vi "Test akwizycji AI Enk.vi"() -> ()   [LabVIEW 2014]
uses:
  <vilib>/DAQmx/create/channels.llb/DAQmx Create Channel (CI-Position-Linear Encoder).vi
  <vilib>/DAQmx/create/channels.llb/DAQmx Create Channel (AI-Voltage-Basic).vi
  <vilib>/DAQmx/configure/timing.llb/DAQmx Timing (Sample Clock).vi
  <vilib>/DAQmx/read.llb/DAQmx Read (Counter 1D DBL 1Chan NSamp).vi
  <vilib>/DAQmx/read.llb/DAQmx Read (Analog 1D Wfm NChan NSamp).vi
panel:
  out "Waveform Graph":waveform(dbl)[](graph)
  in  "error in":errorcluster
  in  "stop":bool
  out "data":dbl[](array[numeric]) format="%#_6p"
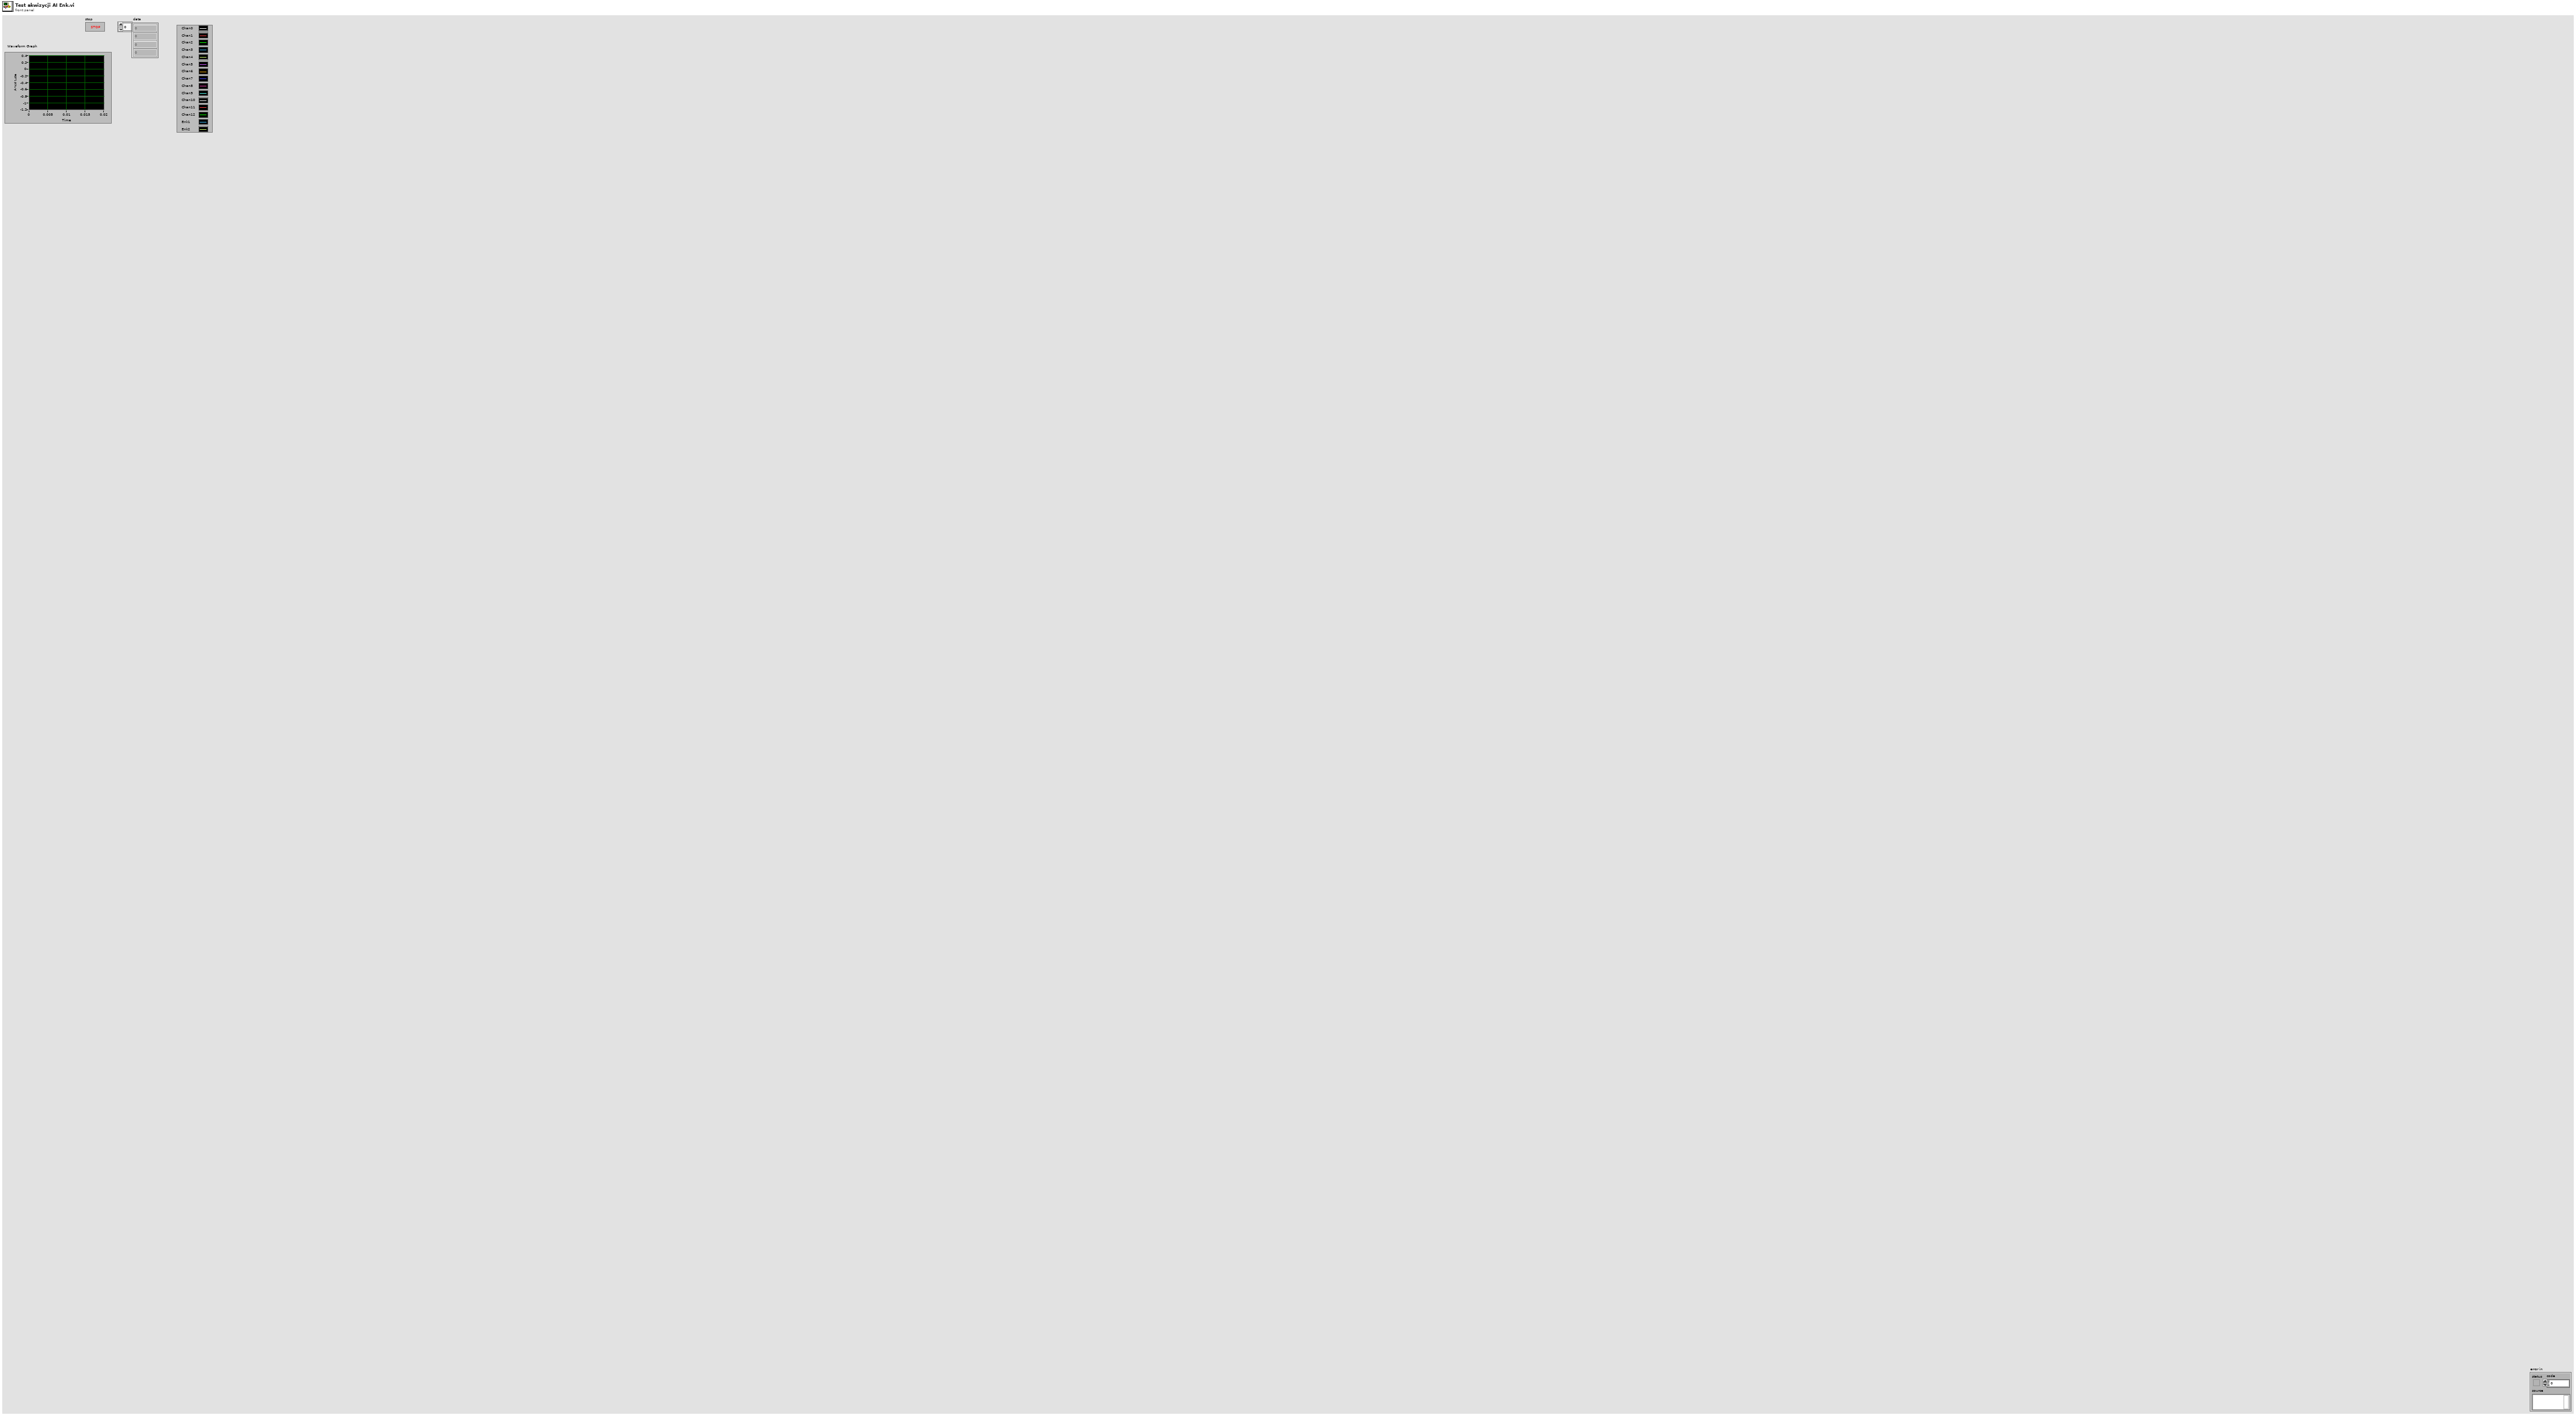
[diagram p1: front panel]
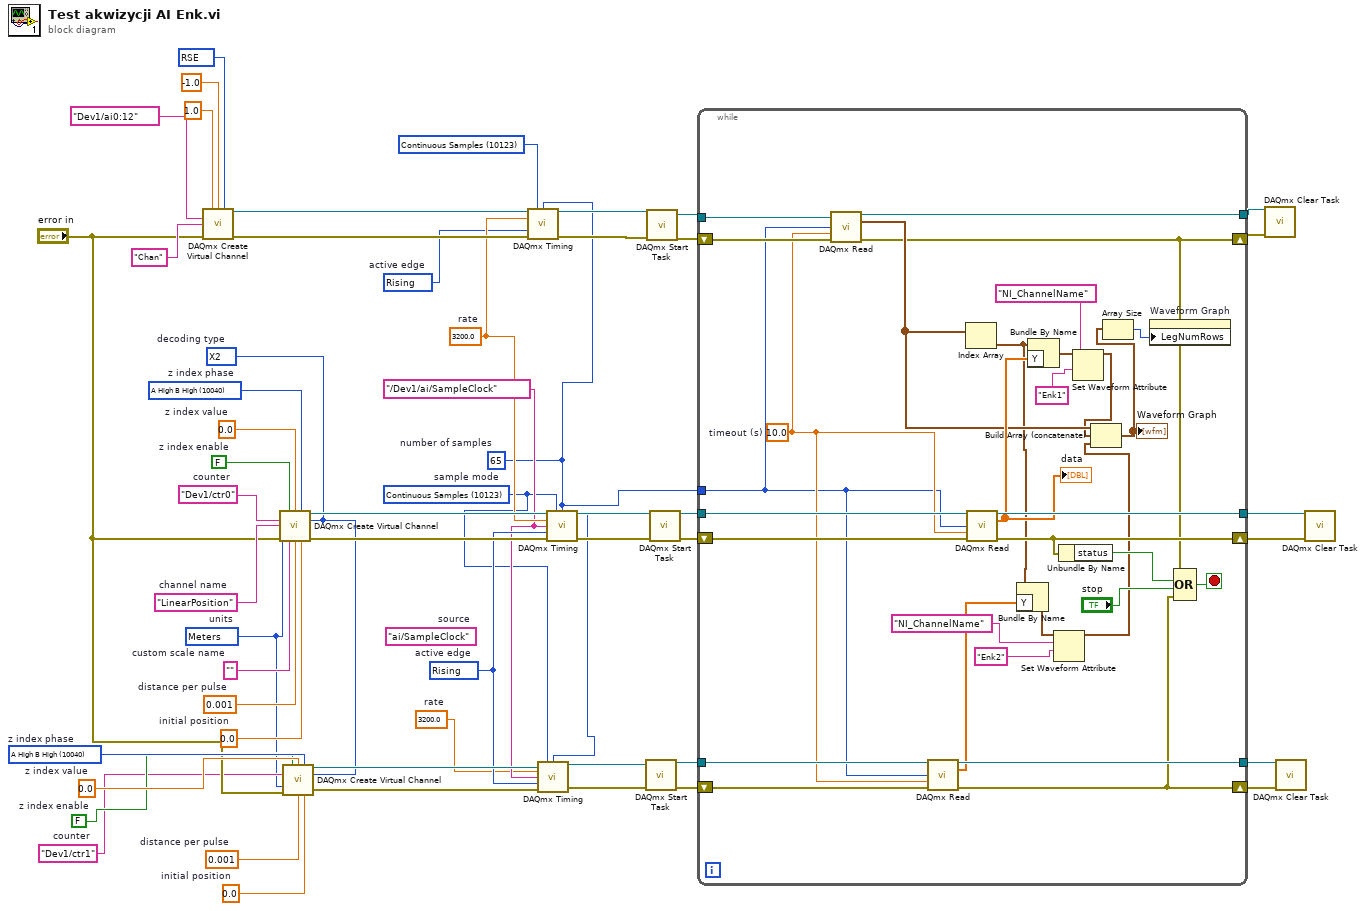
[diagram p0: block diagram]
diagram:
  w5 = 0.0  # initial position
  w6 = 0.001  # distance per pulse
  w12 = 10040 items=["A High B High"=10040, "A High B Low"=10041, "A Low B High"=10042, "A Low B Low"=10043]  # z index phase
  w11 = 0.0  # z index value
  w10 = FALSE  # z index enable
  w8 = "Dev1/ctr1"  # counter
  w15 = 3200.0  # rate
  w25 = 10280 items=["Rising"=10280, "Falling"=10171]  # active edge
  w27 = 10123 items=["Finite Samples"=10178, "Continuous Samples"=10123, "Hardware Timed Single Point"=12522] ("sample mode")
  w16 = tag "/Dev1/ai/SampleClock" ("source")
  w36 = 10083 items=["default"=-1, "RSE"=10083, "NRSE"=10078, "Differential"=10106, "Pseudodifferential"=12529] ("input terminal configuration")
  w13 = 10123 items=["Finite Samples"=10178, "Continuous Samples"=10123, "Hardware Timed Single Point"=12522]  # sample mode
  w26 = 3200.0  # rate
  w17 = 10280 items=["Rising"=10280, "Falling"=10171]  # active edge
  (unwired) "ai/SampleClock"  # source
  w14 = 65  # number of samples
  w7 = 10219 items=["Meters"=10219, "Inches"=10379, "Ticks"=10304, "From Custom Scale"=10065]  # units
  w18 = 10091 items=["X1"=10090, "X2"=10091, "X4"=10092, "Two Pulse Counting"=10313]  # decoding type
  w49 = 0.0  # initial position
  w48 = 0.001  # distance per pulse
  w46 = ""  # custom scale name
  w47 = 10040 items=["A High B High"=10040, "A High B Low"=10041, "A Low B High"=10042, "A Low B Low"=10043]  # z index phase
  w45 = 0.0  # z index value
  w44 = FALSE  # z index enable
  w43 = "LinearPosition"  # channel name
  w41 = "Dev1/ctr0"  # counter
  n1 = call-poly <vilib>:"DAQmx Create Virtual Channel.vi"("maximum value"=1.0, "minimum value"=-1.0, "input terminal configuration"=w36, "physical channels"=tag "Dev1/ai0:12", "name to assign"="Chan", "error in"="error in") -> ("task out"=w28:refnum<k21>, "error out"=w29:errorcluster)  [unwired: 8 in]
  n2 = call-poly <vilib>:"DAQmx Create Virtual Channel.vi"("z index enable"=w44, "z index value"=w45, "z index phase"=w47, "counter"=w41, "decoding type"=w18, "name to assign"=w43, "units"=w7, "error in"="error in", "custom scale name"=w46, "distance per pulse"=w48, "initial position"=w49) -> ("task out"=w50:refnum<k21>, "error out"=w42:errorcluster)  [unwired: 3 in]
  n3 = call-poly <vilib>:"DAQmx Create Virtual Channel.vi"("z index enable"=w10, "z index value"=w11, "z index phase"=w12, "counter"=w8, "decoding type"=w18, "units"=w7, "error in"="error in", "distance per pulse"=w6, "initial position"=w5) -> ("task out"=w22:refnum<k21>, "error out"=w19:errorcluster)  [unwired: 5 in]
  n4 = call-poly <vilib>:"DAQmx Timing.vi"("task/channels in"=w28, "sample mode"=w27, "samples per channel"=w14, "rate"=w26, "active edge"=w25, "error in"=w29) -> ("task out"=w31:refnum<k21>, "error out"=w33:errorcluster)  [unwired: 8 in]
  n5 = call-poly <vilib>:"DAQmx Timing.vi"("task/channels in"=w22, "sample mode"=w13, "samples per channel"=w14, "rate"=w15, "source"=w16, "active edge"=w17, "error in"=w19) -> ("task out"=w21:refnum<k21>, "error out"=w20:errorcluster)  [unwired: 7 in]
  n6 = call-poly <vilib>:"DAQmx Timing.vi"("task/channels in"=w50, "sample mode"=w13, "samples per channel"=w14, "rate"=w26, "source"=w16, "active edge"=w17, "error in"=w42) -> ("task out"=w39:refnum<k21>, "error out"=w40:errorcluster)  [unwired: 7 in]
  n7 = call <vilib>:"DAQmx Start Task.vi"("task/channels in"=w21, "error in"=w20) -> ("task out"=w3:refnum<k21>, "error out"=w4:errorcluster)  [unwired: 12 in]
  n8 = call <vilib>:"DAQmx Start Task.vi"("task/channels in"=w31, "error in"=w33) -> ("task out"=w30:refnum<k21>, "error out"=w32:errorcluster)  [unwired: 12 in]
  n9 = call <vilib>:"DAQmx Start Task.vi"("task/channels in"=w39, "error in"=w40) -> ("task out"=w54:refnum<k21>, "error out"=w53:errorcluster)  [unwired: 12 in]
  n10 = while {
    tunnel: w54 -> [w80]
    tunnel: w14 -> [w65]
    tunnel: [w85] -> w51
    shift-right: [w84] -> w52
    shift-left: w53 -> [w79]
    tunnel: w30 -> [w81]
    shift-right: [w73] -> w24
    shift-left: w32 -> [w82]
    tunnel: [w78] -> w23
    tunnel: w3 -> [w67]
    tunnel: [w64] -> w2
    shift-right: [w63] -> w1
    shift-left: w4 -> [w68]
    stop <- w74 stop-if-true
    w66 = 10.0  # timeout (s)
    n11 = call-poly <vilib>:"DAQmx Read.vi"("task/channels in"=w81, "number of samples per channel"=w65, "timeout"=w66, "error in"=w82) -> ("task out"=w78:refnum<k21>, "data"=w77:waveform(dbl)[], "error out"=w73:errorcluster)  [unwired: 9 in]
    n12 = call-poly <vilib>:"DAQmx Read.vi"("task/channels in"=w67, "number of samples per channel"=w65, "timeout"=w66, "error in"=w68) -> ("task out"=w64:refnum<k21>, "data"=w60:dbl[], "error out"=w63:errorcluster)  [unwired: 9 in]
    n13 = Index Array(array=w77) -> (element=w61:waveform(dbl))  [unwired: 1 in]
    n14 = call-poly <vilib>:"DAQmx Read.vi"("task/channels in"=w80, "number of samples per channel"=w65, "timeout"=w66, "error in"=w79) -> ("task out"=w85:refnum<k21>, "data"=w83:dbl[], "error out"=w84:errorcluster)  [unwired: 9 in]
    "data" <- w83
    n15 = Bundle By Name(cluster=w61, "Y"=w60) -> (w62:waveform(dbl))
    n16 = Bundle By Name(cluster=w61, "Y"=w83) -> (w72:waveform(dbl))
    n17 = Set Waveform Attribute(5:"Enk2" ("name"), 6:"NI_ChannelName" ("name"), 7:w62) -> (3:w59:waveform(dbl))  [unwired: 1 in, 2 out]
    n18 = Unbundle By Name(w84) -> ("status"=w75:bool)
    n19 = Set Waveform Attribute(5:"Enk1" ("name"), 6:"NI_ChannelName" ("name"), 7:w72) -> (3:w71:waveform(dbl))  [unwired: 1 in, 2 out]
    n20 = Build Array (concatenate)(w77, w71, w59) -> (w55:waveform(dbl)[])
    "Waveform Graph" <- w55
    n21 = Array Size(array=w55) -> (size(s)=w56:i32)
    n22 = property on="Waveform Graph" class="WFGraph (strict)"("LegNumRows"=w56) -> ()  [unwired: 2 in, 2 out]
    n23 = Compound Arithmetic op=OR(w73, w75, "stop", w63) -> (w74:bool)
  }
  n24 = call <vilib>:"DAQmx Clear Task.vi"("task in"=w23, "error in"=w24) -> ()  [unwired: 13 in, 1 out]
  n25 = call <vilib>:"DAQmx Clear Task.vi"("task in"=w2, "error in"=w1) -> ()  [unwired: 13 in, 1 out]
  n26 = call <vilib>:"DAQmx Clear Task.vi"("task in"=w51, "error in"=w52) -> ()  [unwired: 13 in, 1 out]
